vi "HART_Address.vi"(7 "Primary Master":u8=138 format="%.0x", 10 "Tag no. (device ID)":u32=11362001 format="%.0x", 11 "Dev Type":u8=63 format="%.0x") -> (2 "Address":u8[](array[numeric]) format="%.0x")   [LabVIEW 2016]
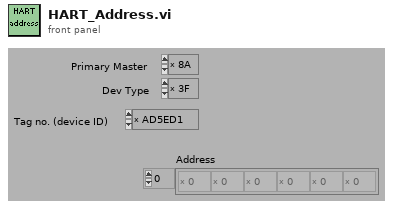
[diagram p1: front panel]
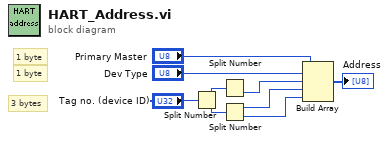
[diagram p0: block diagram]
diagram:
  # "1 byte"
  # "1 byte"
  # "3 bytes"
  n1 = Split Number(x="Tag no. (device ID)") -> (hi(x)=w9:u16, lo(x)=w8:u16)
  n2 = Split Number(x=w9) -> (lo(x)=w5:u8)  [unwired: 1 out]
  n3 = Split Number(x=w8) -> (hi(x)=w4:u8, lo(x)=w3:u8)
  n4 = Build Array("Primary Master", "Dev Type", w5, w4, w3) -> (→"Address":u8[])
